vi "Colse port.vi"(8 "error in (no error)":errorcluster, 11 "Serial in":refnum<class "Serial.lvclass">) -> (0 "error out":errorcluster)   [LabVIEW 2019, in "Serial.lvclass"]
uses:
  Serial.lvclass
  Serial.lvclass/Serial.ctl
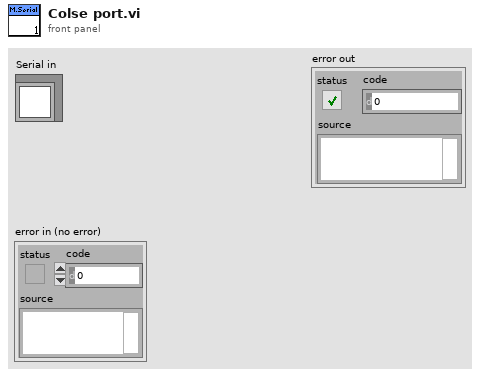
[diagram p1: front panel]
types:
  T1 = typedef "Semaphore RefNum" = refnum<k1>
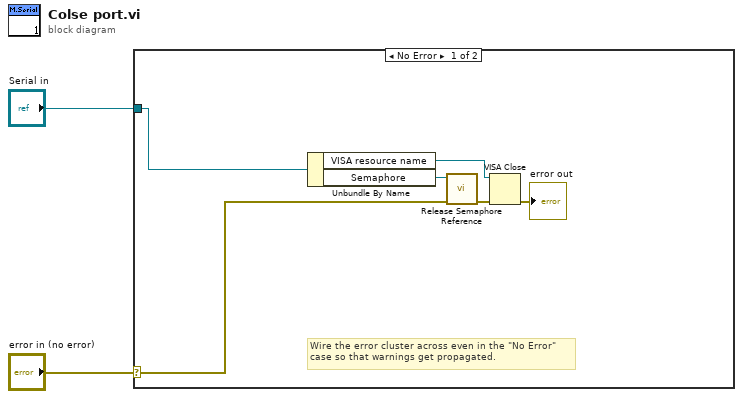
[diagram p0: block diagram]
diagram:
  n1 = case shown="No Error" "error in (no error)" {
    selector: "error in (no error)" -> [w4 _]
    tunnel: "Serial in" -> [w5 _]
    frame No Error {
      # "Wire the error cluster across even in the \"No Error\"\ncase so that warnings get propagated."
      n2 = Unbundle By Name(w5) -> ("VISA resource name"=w8:refnum<visa-resource-name>, "Semaphore"=w7:T1)
      n3 = call <vilib>:"Release Semaphore Reference.vi"("error in (no error)"=w4, "semaphore"=w7) -> ("error out"=w6:errorcluster)  [unwired: 8 in, 1 out]
      n4 = VISA Close(VISA resource name=w8, error in (no error)=w6) -> (error out=→"error out":errorcluster)
    }
    frame Error {
    }
  }
